vi "exercice_8-2.vi"() -> ()   [LabVIEW 2013]
uses:
  <vilib>/DAQmx/read.llb/DAQmx Read (Analog DBL 1Chan 1Samp).vi
  <vilib>/DAQmx/miscellaneous.llb/DAQmx Fill In Error Info.vi
  <vilib>/ptbypt/NI_PtbyPt.lvlib
panel:
  out "Graphe":cluster{"mean":dbl, "data":dbl}(graph)
  out "Tableau":dbl[](array[numeric])
  out "data":dbl caption="données" format="%0.2f"
  in  "stop":bool
  in  "Nom de tâche DAQmx":refnum<k21>
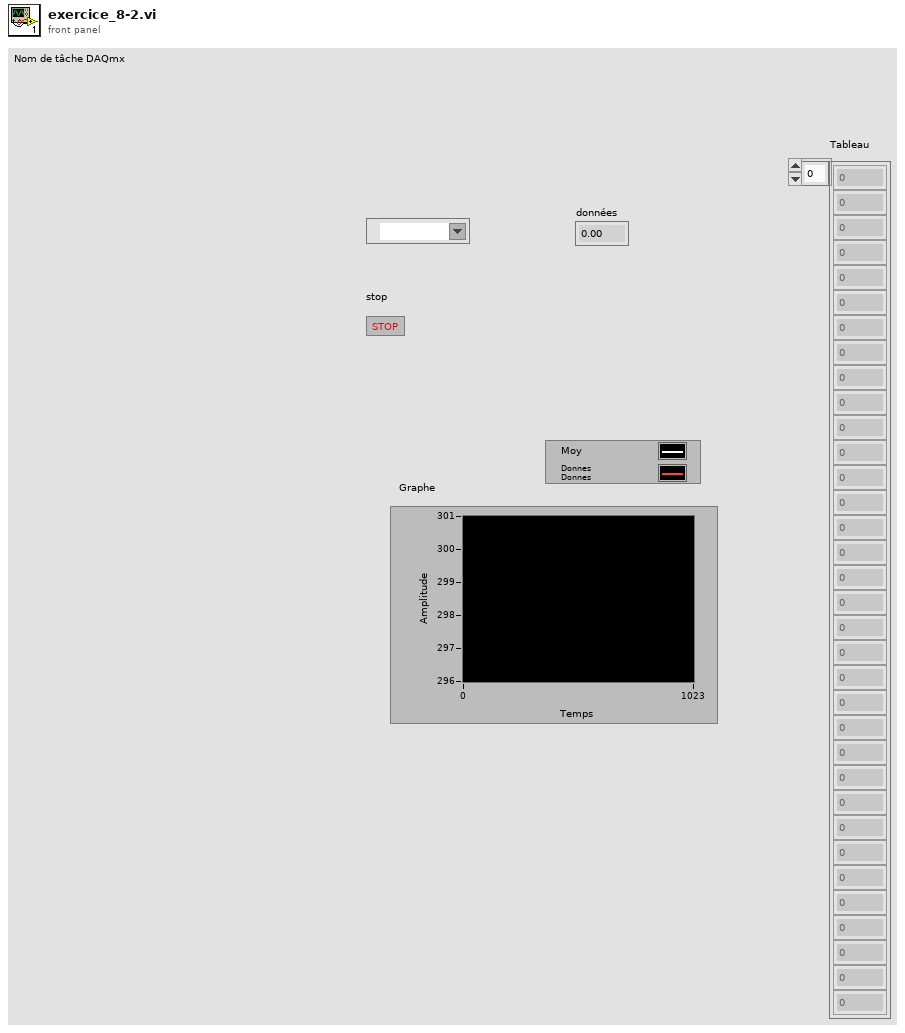
[diagram p1: front panel]
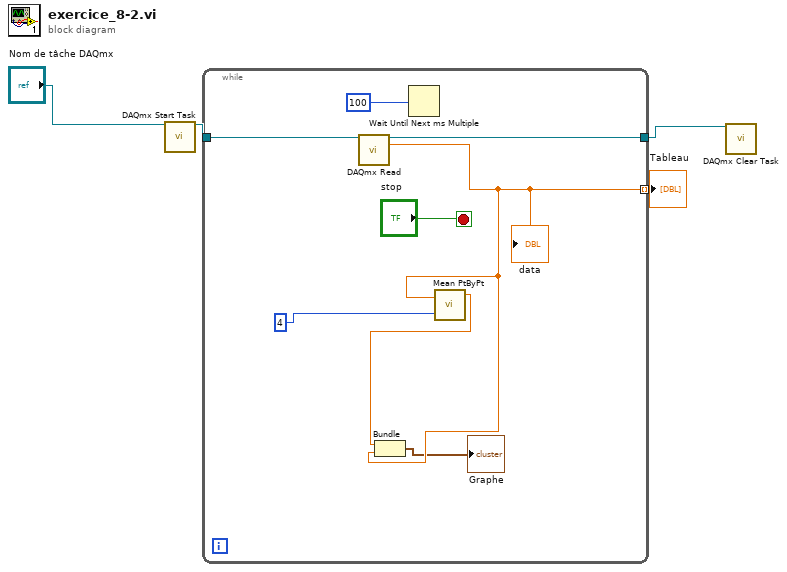
[diagram p0: block diagram]
diagram:
  n1 = call <vilib>:"DAQmx Start Task.vi"("task/channels in"="Nom de tâche DAQmx") -> ("task out"=w3:refnum<k21>)  [unwired: 13 in, 1 out]
  n2 = while {
    tunnel: w3 -> [w12]
    tunnel: [w11] -> w2
    tunnel: [w6] -> w1 mode=indexing
    stop <- "stop" stop-if-true
    n3 = call-poly <vilib>:"DAQmx Read.vi"("task/channels in"=w12) -> ("task out"=w11:refnum<k21>, "data"=w6:dbl)  [unwired: 12 in, 1 out]
    "data" <- w6
    n4 = Wait Until Next ms Multiple(millisecond multiple=100) -> ()  [unwired: 1 out]
    n5 = call <vilib>:"Mean PtByPt.vi"("x"=w6, "sample length"=4) -> ("mean"=w7:dbl)  [unwired: 2 in, 1 out]
    n6 = Bundle("mean"=w7, "data"=w6) -> (→"Graphe":cluster{"mean":dbl, "data":dbl})  [unwired: 1 in]
  }
  "Tableau" <- w1
  n7 = call <vilib>:"DAQmx Clear Task.vi"("task in"=w2) -> ()  [unwired: 14 in, 1 out]
